vi "ParameterDelete.vi"(7 "productsName":string, 11 "parameterName":string) -> ()   [LabVIEW 2012]
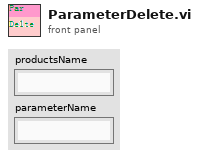
[diagram p1: front panel]
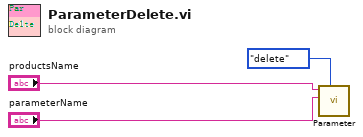
[diagram p0: block diagram]
diagram:
  n1 = call "Parameter.vi"("模式"=enum16{"select", "insert", "update", "delete"}."delete", "parameterName"="parameterName", "productsName"="productsName") -> ()  [unwired: 8 in, 1 out]
